vi "调用文件处理子vi例子.vi"() -> ()   [LabVIEW 2023]
panel:
  out "error constant":errorcluster
  out "String":string
  in  "file path (use dialog)":path
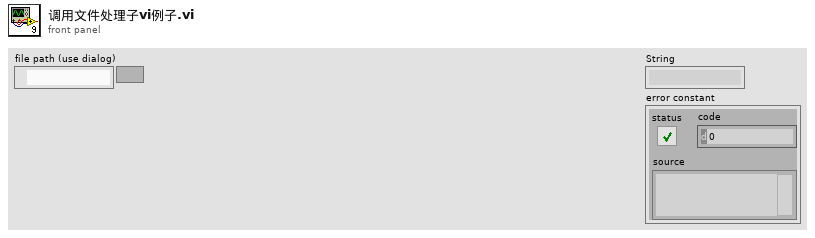
[diagram p1: front panel]
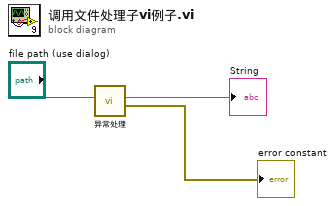
[diagram p0: block diagram]
diagram:
  n1 = call "异常处理.vi"("file path (use dialog)"="file path (use dialog)") -> ("error constant"=→"error constant":errorcluster, "String"=→"String":string)  [unwired: 9 in]
